vi "Read epoll fd.vi"(8 "error in (no error)":errorcluster, 11 "Unix Pipe Reader in":refnum<class "Unix Pipe Reader.lvclass">) -> (0 "error out":errorcluster, 2 "epoll fd":i32, 3 "Unix Pipe Reader out":refnum<class "Unix Pipe Reader.lvclass">)   [LabVIEW 2013, in "Linux RT IPC.Pipes.lvlib" / "Unix Pipe Reader.lvclass"]
uses:
  Unix Pipe Reader.lvclass
  Unix Pipe Reader.lvclass/Unix Pipe Reader.ctl
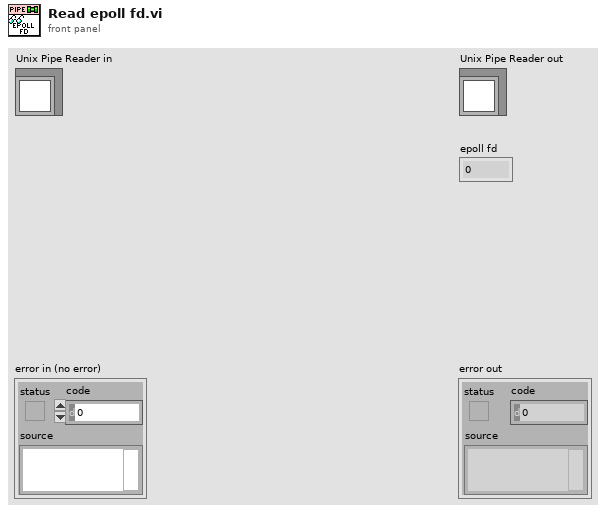
[diagram p1: front panel]
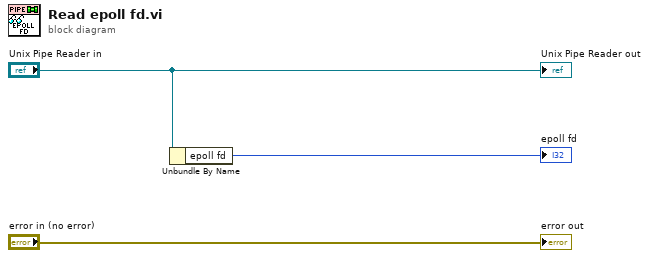
[diagram p0: block diagram]
diagram:
  n1 = Unbundle By Name("Unix Pipe Reader in") -> ("epoll fd"=→"epoll fd":i32)
  "error out" <- "error in (no error)"
  "Unix Pipe Reader out" <- "Unix Pipe Reader in"
